vi "Generate Sweep folder.vi"(8 "error in (no error)":errorcluster) -> (0 "error out":errorcluster, 3 "Timelapse folder path":path)   [LabVIEW 2017]
uses:
  Typedefs/Experiment folder base name.ctl
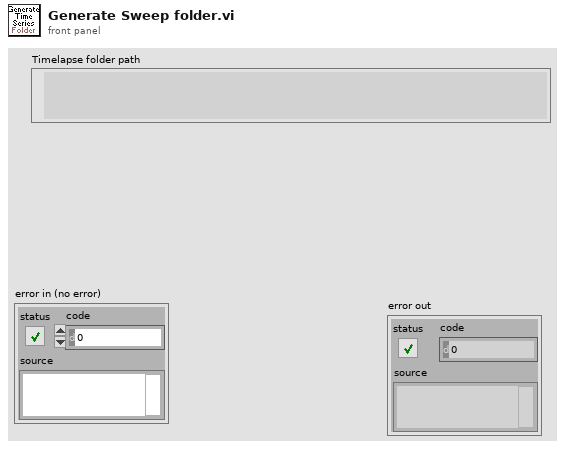
[diagram p1: front panel]
types:
  T1 = typedef "Experiment folder base name.ctl" = enum16{"TimeLapse", "FunctAcq", "ParSweep"}
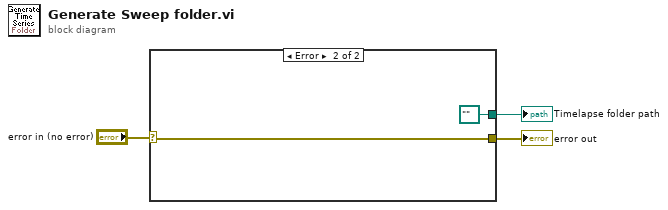
[diagram p0: block diagram]
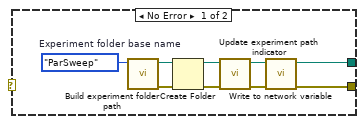
[diagram p2: hidden frame]
diagram:
  n1 = case shown="Error" "error in (no error)" {
    selector: "error in (no error)" -> [_ w14]
    tunnel: [w12 w14] -> w3
    tunnel: [w11 path "" ("created path (dup)")] -> w1
    frame No Error {
      w4 = Experiment_folder_base_name."ParSweep"  # Experiment folder base name
      n2 = call "Build experiment folder path.vi"("Experiment folder base name"=w4) -> ("error out"=w6:errorcluster, "Experiment folder  file path"=w8:path)  [unwired: 9 in]
      n3 = Create Folder(path (use dialog)=w8, error in=w6) -> (created path=w7:path, error out=w5:errorcluster)  [unwired: 1 in, 1 out]
      n4 = call "Update experiment path indicator.vi"("error in (no error)"=w5, "created path"=w7) -> ("error out"=w9:errorcluster, "created path (dup)"=w10:path)  [unwired: 8 in]
      n5 = call "Write to network variable.vi"("error in (no error)"=w9, "created path"=w10) -> ("error out"=w12:errorcluster, "created path (dup)"=w11:path)  [unwired: 8 in]
    }
    frame Error {
    }
  }
  "Timelapse folder path" <- w1
  "error out" <- w3
